vi "Get Typed Value.vi"(7 "Type":refnum<class>, 8 "error in (no error)":errorcluster, 11 "PathTreeNode in":refnum<class "PathTreeNode.lvclass">) -> (0 "error out":errorcluster, 2 "Typed Value":refnum<class>, 3 "PathTreeNode out":refnum<class "PathTreeNode.lvclass">)   [LabVIEW 2020, in "Advanced Structures.lvlib" / "PathTreeNode.lvclass"]
uses:
  PathTreeNode.lvclass
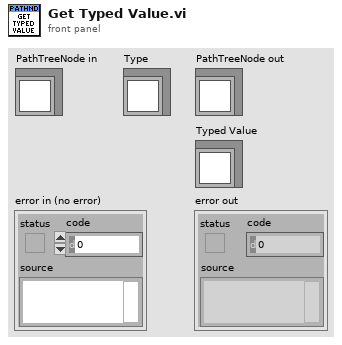
[diagram p1: front panel]
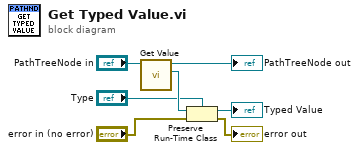
[diagram p0: block diagram]
diagram:
  n1 = call "Get Value.vi"("PathTreeNode in"="PathTreeNode in") -> ("Value"=w5:refnum<class>, "PathTreeNode out"=→"PathTreeNode out":refnum<class "PathTreeNode.lvclass">)  [unwired: 8 in, 1 out]
  n2 = Preserve Run-Time Class(object in=w5, error in="error in (no error)", 2:"Type") -> (object out=→"Typed Value":refnum<class>, error out=→"error out":errorcluster)
